vi "PH_SHS_Analysis.set modified data.vi"(0 "i ref in":refnum<vi>, 2 "i attribute":T1={"GUI Refs"={"Delete"=refnum, "Global On"=refnum, "Cam Source"=refnum, "Calibration Data File"=refnum, "Calibration status"=refnum, "Show overlay"=refnum, "SHS Device Config"=refnum, "Result"=refnum, "Consider Tilt"=refnum, "Working Reference"=refnum, "Remove Tilt"=refnum, "Take Cali  Reference"=refnum, "Publishing Data Status"=refnum, "Calibration Data"=refnum}, "Calibration"={"Status"=0, "Data"={"Date"="", "Time"="", "Cam Settings"={"Cam ID"="", "Gain"=0.0, "Brightness"=0.0, "Shutter"=0.0, "Cam Error"=FALSE, "Mode"=0}, "SHS Reference Result"={"Reference"=[], "Lens Array Pitch [px]"=0.0}, "Pixel Size"=0.0, "MLA Pitch"=0.0, "Method"=enum."automatic", "Calibration Data calculated"=FALSE, "No Problems at calculation?"=FALSE, "error out"={"status"=FALSE, "code"=0, "source"=""}}, "File"=path ""}, "Result"={"Time Stamp"=timestamp(0 s since 1904-01-01), "Zernike Coefficients"={"Tilt x"=0.0, "Tilt y"=0.0, "Defocus"=0.0, "Astig 0°"=0.0, "Astig 45°"=0.0, "Coma x"=0.0, "Coma y"=0.0, "Spherical"=0.0, "Trefoil 0°"=0.0, "Trefoil 30°"=0.0, "2nd Astig 0°"=0.0, "2nd Astig 45°"=0.0, "2nd Coma x"=0.0, "2nd Coma y"=0.0, "2nd Spherical"=0.0}, "PtV [lambda]"=0.0, "Shifts"=[], "Measurement Quality"={0.0, 0.0, 0.0}, "Measurement valid?"=FALSE}, "Image"=refnum, "SHS Device Config"={"focal length [m]"=0.01, "pixel size [m/px]"=6.7e-06, "wavelength [m]"=1.053e-06}, "Show Overlay"=FALSE, "GradientZernikeMatrix"=[], "Consider Tilt"=FALSE, "Working Reference"={"Reference"=[], "Lens Array Pitch [px]"=0.0}, "Zernicke Service ID"=-1, "PSDB Image"=refnum} {"SHS Device Config"."wavelength [m]" format="%#_6p"; "SHS Device Config"."pixel size [m/px]" format="%#_6p"; "SHS Device Config"."focal length [m]" format="%#_6p"; "Result"."Measurement Quality" scale=0.0..12.0; "Result"."Zernike Coefficients"."2nd Spherical" scale=-2.0..2.0 scale format="%.2f"; "Result"."Zernike Coefficients"."2nd Coma y" scale=-2.0..2.0 scale format="%.2f"; "Result"."Zernike Coefficients"."2nd Coma x" scale=-2.0..2.0 scale format="%.2f"; "Result"."Zernike Coefficients"."2nd Astig 45°" scale=-2.0..2.0 scale format="%.2f"; "Result"."Zernike Coefficients"."2nd Astig 0°" scale=-2.0..2.0 scale format="%.2f"; "Result"."Zernike Coefficients"."Trefoil 30°" scale=-2.0..2.0 scale format="%.2f"; "Result"."Zernike Coefficients"."Trefoil 0°" scale=-2.0..2.0 scale format="%.2f"; "Result"."Zernike Coefficients"."Spherical" scale=-2.0..2.0 scale format="%.2f"; "Result"."Zernike Coefficients"."Coma y" scale=-2.0..2.0 scale format="%.2f"; "Result"."Zernike Coefficients"."Coma x" scale=-2.0..2.0 scale format="%.2f"; "Result"."Zernike Coefficients"."Astig 45°" scale=-2.0..2.0 scale format="%.2f"; "Result"."Zernike Coefficients"."Astig 0°" scale=-2.0..2.0 scale format="%.2f"; "Result"."Zernike Coefficients"."Defocus" scale=-2.0..2.0 scale format="%.2f"; "Result"."Zernike Coefficients"."Tilt y" scale=-2.0..2.0 scale format="%.2f"; "Result"."Zernike Coefficients"."Tilt x" scale=-2.0..2.0 scale format="%.2f"; "Result"."Time Stamp" format="%<%H:%M:%S%2u\n%y/%m/%d>T"; "Calibration"."Status" items=["no info", "off/false/out", "on/true/in", "Failure", "Alarm", "Status 1", "Status 2", "Status 3"]}, 5 "error in (no error)":errorcluster) -> (14 "i ref out":refnum<vi>, 19 "error out":errorcluster)   [LabVIEW 2014, in "PH_SHS_Analysis.lvlib"]
doc: "Writes the data into the attribute of an object. Then, the attribute dara are unlocked using the \"release\" method. Prior to calling THIS method, the attribute data must have been locked using the methods \"lock\" or \"get data to modify\".\n\n\nLicense Agreement for this software:\n\nCopyright (C)\nGesellschaft für Schwerionenforschung, GSI\nPlanckstr. 1\n64291 Darmstadt\nGermany\n\nContact: D.Beck@gsi.de \n\nThis program is free software; you can redistribute it and/or modify it under the terms of the GNU General Public License as published by the Free Software Foundation; either version 2 of the license, or (at your option) any later version.\n\nThis program is distributed in the hope that it will be useful, but WITHOUT ANY WARRANTY; without even the implied warranty of MERCHANTABILITY or FITNESS FOR A PARTICULAR PURPOSE. See the GNU General License for more details (http://www.gnu.org).\n\nGesellschaft für Schwerionenforschung, GSI\nPlanckstr. 1, 64291 Darmstadt, Germany\nFor all questions and ideas contact: M.Richter@gsi.de, H.Brand@gsi.de or D.Beck@gsi.de.\nLast update: 17-JUN-2004"
uses:
  PH_SHS_Analysis.lvlib
  PH_SHS_Analysis.i attribute.ctl
  PH_Basics/PH_StatusHandler/PH_StatusHandler.Status.ctl
  PH_SHS_Analysis_Calibrator/PH_SHS_Analysis_Calibrator.Analysis Calibration Data.ctl
  CSlibraries-extern/shs/SHS_Common/SHSReference.ctl
  CSlibraries-extern/shs/SHS_Common/ReferencePoint.ctl
  CSlibraries-extern/shs/SHS_Common/Rectangle.ctl
  CSlibraries-extern/shs/SHS_Common/Point.ctl
  PH_SHS_Analysis.Result.ctl
  PH_SHS_Analysis.Zernike Coefficients.ctl
  CSlibraries-extern/shs/SHS_Common/Shifts.ctl
  <vilib>/vision/Image Controls.llb/IMAQ Image.ctl
  CSlibraries-extern/shs/SHS_Analysis/SHS_DeviceConfig.ctl
  CS_Core/CSObj/CSObj.lvlib
  CSlibraries-extern/shs/SHS_Common/SHS_Common.lvlib
  PH_SHS_Analysis_Calibrator/PH_SHS_Analysis_Calibrator.lvlib
  CSlibraries-extern/shs/SHS_Analysis/SHS_Analysis.lvlib
  PH_Basics/PH_StatusHandler/PH_StatusHandler.lvlib
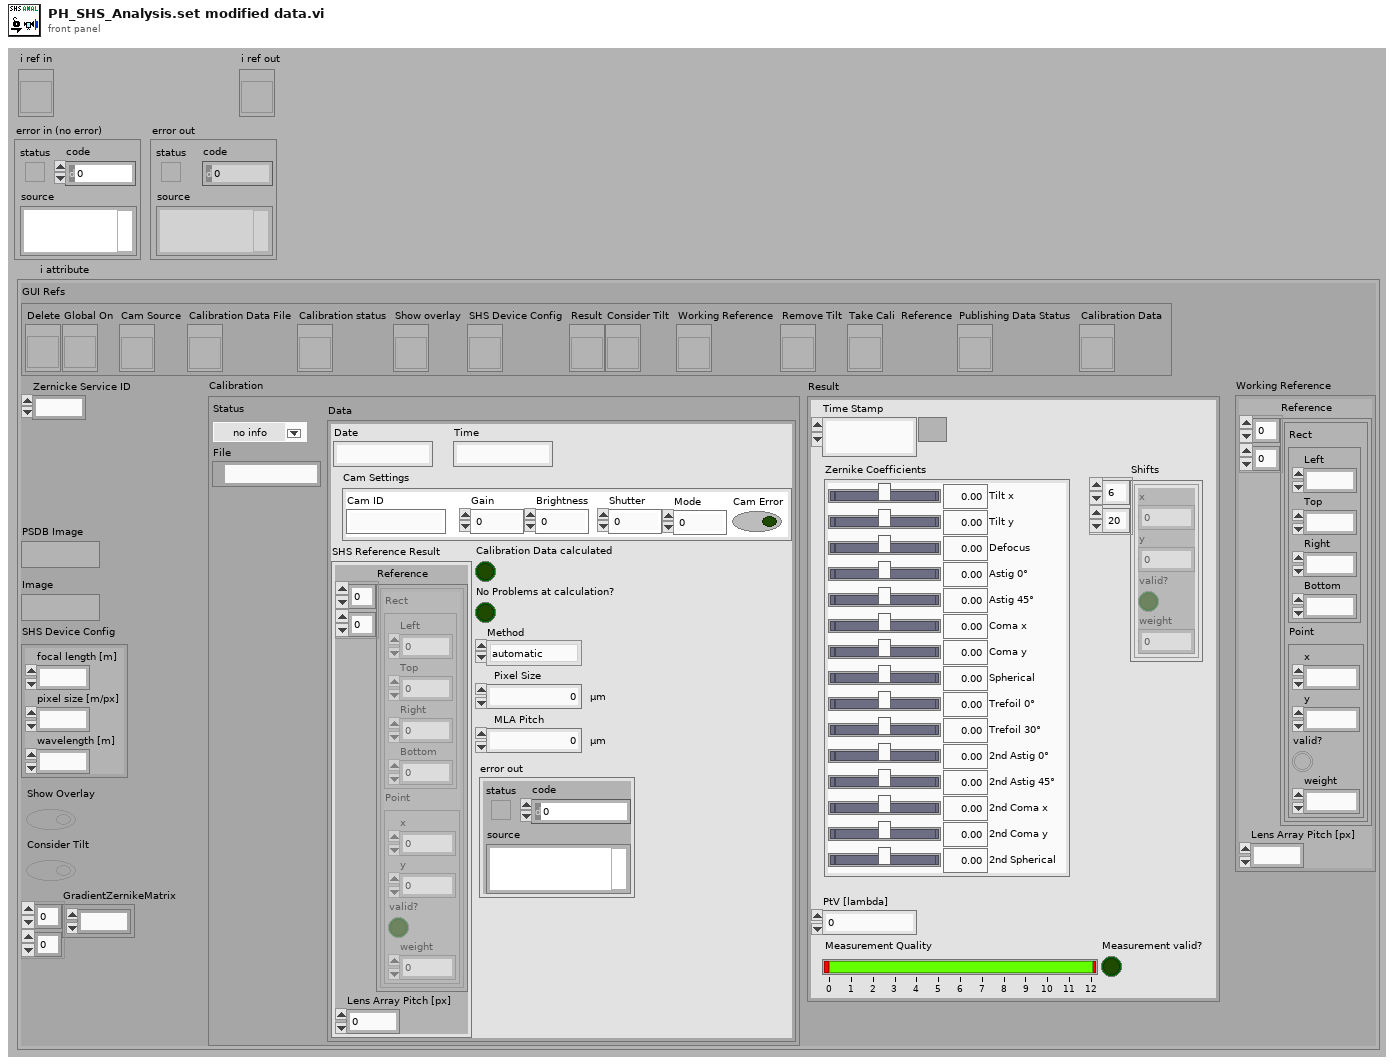
[diagram p1: front panel]
types:
  T1 = typedef "PH_SHS_Analysis.lvlib/PH_SHS_Analysis.i attribute.ctl" = cluster{"GUI Refs":cluster{"Delete":refnum<vi>, "Global On":refnum<vi>, "Cam Source":refnum<vi>, "Calibration Data File":refnum<vi>, "Calibration status":refnum<vi>, "Show overlay":refnum<vi>, "SHS Device Config":refnum<vi>, "Result":refnum<vi>, "Consider Tilt":refnum<vi>, "Working Reference":refnum<vi>, "Remove Tilt":refnum<vi>, "Take Cali  Reference":refnum<vi>, "Publishing Data Status":refnum<vi>, "Calibration Data":refnum<vi>}, "Calibration":cluster{"Status":T2, "Data":T3, "File":path}, "Result":T8, "Image":T11, "SHS Device Config":T12, "Show Overlay":bool, "GradientZernikeMatrix":dbl[][], "Consider Tilt":bool, "Working Reference":T4, "Zernicke Service ID":i32, "PSDB Image":T11}
  T2 = typedef "PH_StatusHandler.lvlib/PH_StatusHandler.Status.ctl" = i16
  T3 = typedef "PH_SHS_Analysis_Calibrator.lvlib/PH_SHS_Analysis_Calibrator.Analysis Calibration Data.ctl" = cluster{"Date":string, "Time":string, "Cam Settings":cluster{"Cam ID":string, "Gain":dbl, "Brightness":dbl, "Shutter":dbl, "Cam Error":bool, "Mode":i32}, "SHS Reference Result":T4, "Pixel Size":dbl, "MLA Pitch":dbl, "Method":enum16{"automatic", "manual"}, "Calibration Data calculated":bool, "No Problems at calculation?":bool, "error out":errorcluster}
  T4 = typedef "SHS_Common.lvlib/SHSReference.ctl" = cluster{"Reference":T5[][], "Lens Array Pitch [px]":dbl}
  T5 = typedef "SHS_Common.lvlib/ReferencePoint.ctl" = cluster{"Rect":T6, "Point":T7}
  T6 = typedef "SHS_Common.lvlib/Rectangle.ctl" = cluster{"Left":i32, "Top":i32, "Right":i32, "Bottom":i32}
  T7 = typedef "SHS_Common.lvlib/Point.ctl" = cluster{"x":dbl, "y":dbl, "valid?":bool, "weight":dbl}
  T8 = typedef "PH_SHS_Analysis.lvlib/PH_SHS_Analysis.Result.ctl" = cluster{"Time Stamp":timestamp, "Zernike Coefficients":T9, "PtV [lambda]":dbl, "Shifts":T10, "Measurement Quality":cluster{dbl, dbl, dbl}, "Measurement valid?":bool}
  T9 = typedef "PH_SHS_Analysis.lvlib/PH_SHS_Analysis.Zernike Coefficients.ctl" = cluster{"Tilt x":dbl, "Tilt y":dbl, "Defocus":dbl, "Astig 0°":dbl, "Astig 45°":dbl, "Coma x":dbl, "Coma y":dbl, "Spherical":dbl, "Trefoil 0°":dbl, "Trefoil 30°":dbl, "2nd Astig 0°":dbl, "2nd Astig 45°":dbl, "2nd Coma x":dbl, "2nd Coma y":dbl, "2nd Spherical":dbl}
  T10 = typedef "SHS_Common.lvlib/Shifts.ctl" = T7[][]
  T11 = typedef "IMAQ Image.ctl" = refnum<image>
  T12 = typedef "SHS_Analysis.lvlib/SHS_DeviceConfig.ctl" = cluster{"focal length [m]":dbl, "pixel size [m/px]":dbl, "wavelength [m]":dbl}
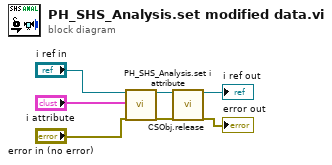
[diagram p0: block diagram]
diagram:
  n1 = call "PH_SHS_Analysis.set i attribute.vi"("i ref in"="i ref in", "i attribute"="i attribute", "error in (no error)"="error in (no error)") -> ("i ref out"=w4:refnum<vi>, "error out"=w3:errorcluster)  [unwired: 15 in]
  n2 = call "CSObj.release.vi"("i ref in"=w4, "error in (no error)"=w3) -> ("i ref out"=→"i ref out":refnum<vi>, "error out"=→"error out":errorcluster)  [unwired: 16 in]
